vi "TTM.vi"() -> ()   [LabVIEW 2019]
doc: "This is the Target Temperature Monitoring module (TTM).\nIts job is to read all temperature measurement devices and report back the information."
uses:
  TTM Global.vi
panel:
  out "status_THCD401":bool
  in  "port_THCD401":u16=10003
  in  "addr_THCD401":string="192.168.24.17"
  in  "read_flow":bool=TRUE caption="Read Flow"
  out "status_1000":bool
  in  "port_1000":u16=10001
  out "status_He3":bool
  in  "port_He3":u16=10002
  in  "addr_He3":string="192.168.24.17"
  in  "port":u16=10000
  in  "addr":string="192.168.24.17"
  out "status":bool
  in  "Read LakeShore":bool
  in  "Read ITC4":bool
  in  "Read He4 Manometer":bool=TRUE
  in  "Read He3 Manometer":bool
  in  "He4 Range":enum32{"X 1", "X 0.1", "X 0.01", "X 0.001"}(ring)=enum."X 0.01"
  in  "He3 Range":i32(ring)=2 items=["range X0.01", "range X0.1", "range X1"]
  out "TTM Message Type":T1(ring)=enum."He3Range="
  # "He4:100"
  # "He4:1000"
  # "He3"
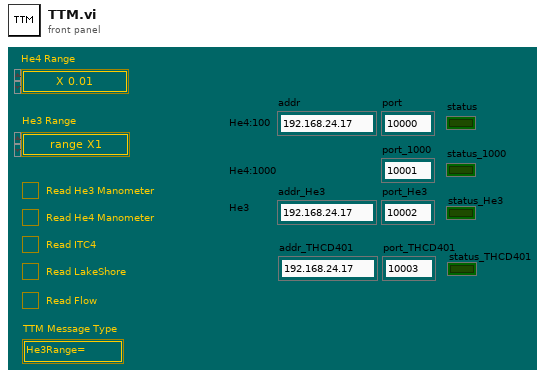
[diagram p1: front panel]
types:
  T1 = enum16{"No Message", "Bad Message", "He3Range=", "He4Range=", "GenEvent=", "Ping=", "Stop"}
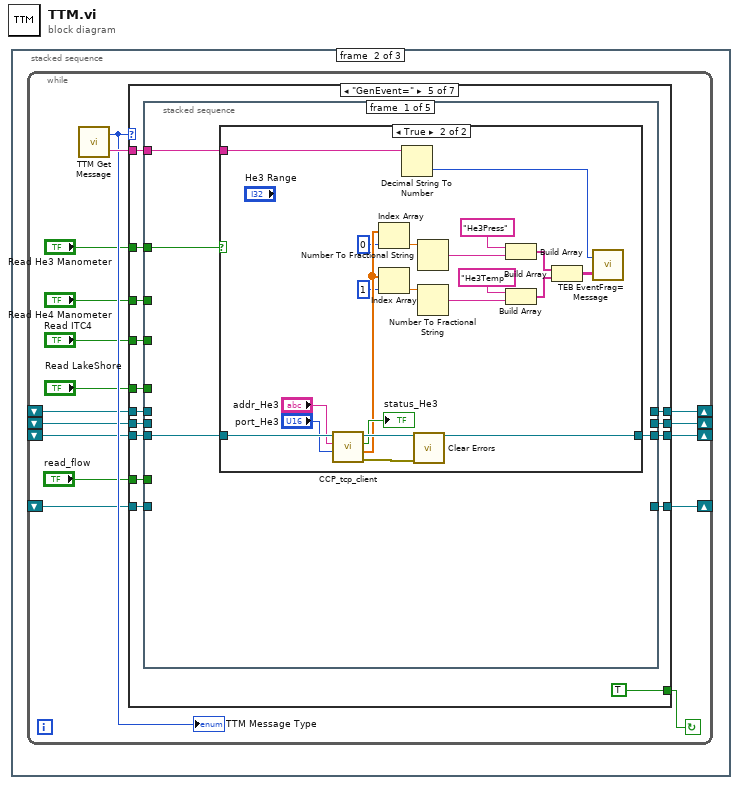
[diagram p0: block diagram]
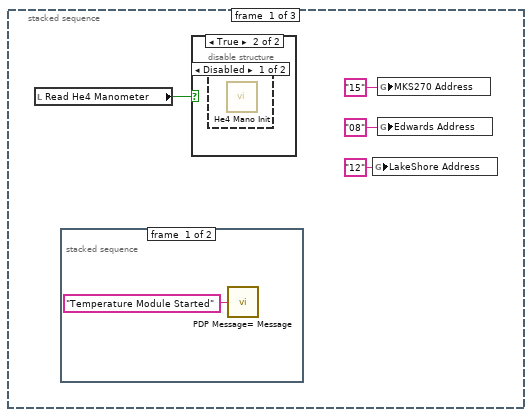
[diagram p2: hidden frame]
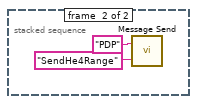
[diagram p5: hidden frame]
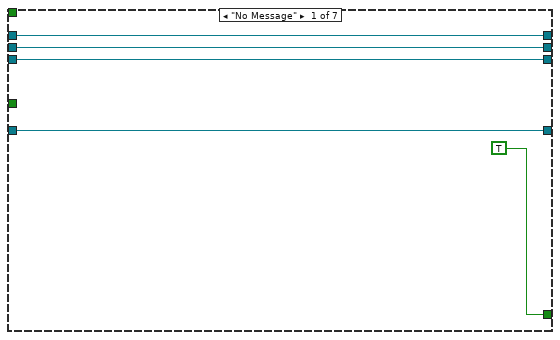
[diagram p6: hidden frame]
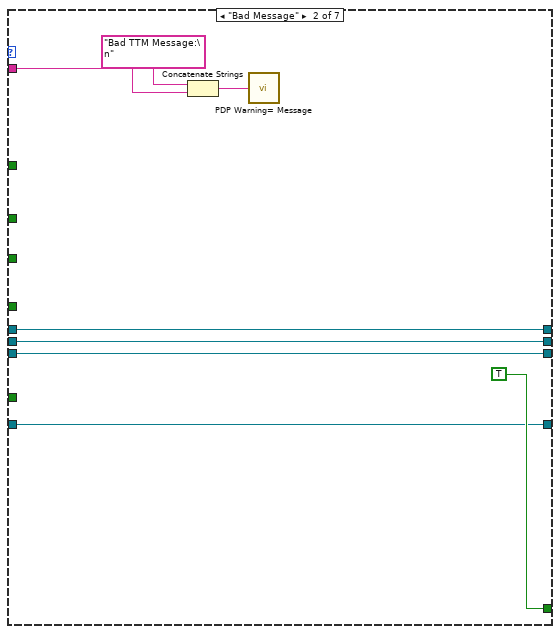
[diagram p7: hidden frame]
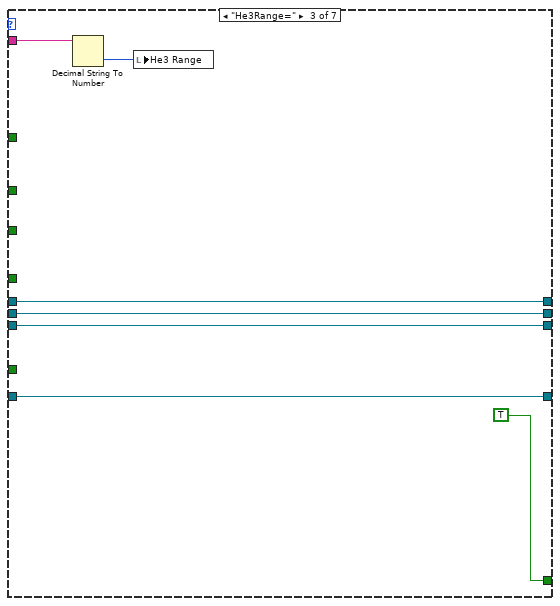
[diagram p8: hidden frame]
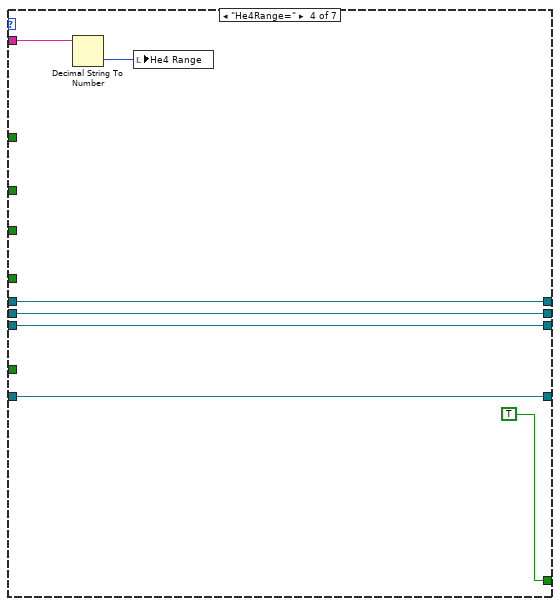
[diagram p9: hidden frame]
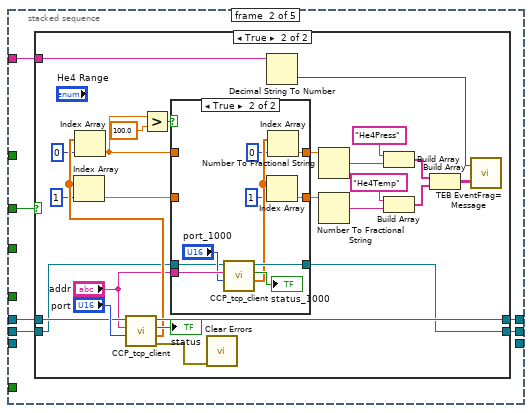
[diagram p11: hidden frame]
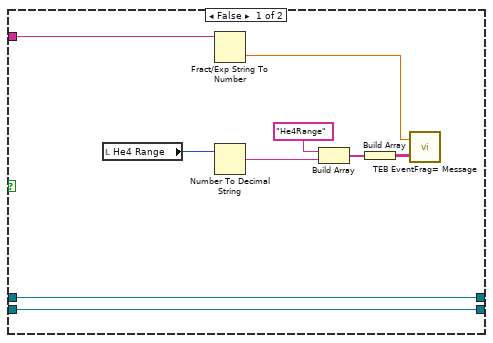
[diagram p12: hidden frame]
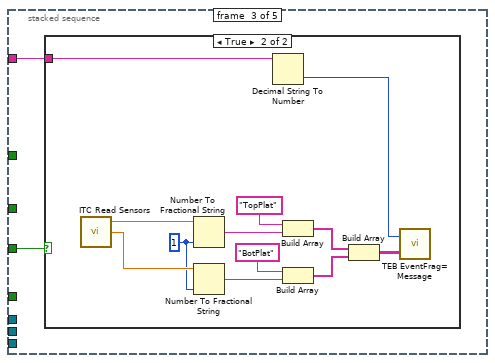
[diagram p14: hidden frame]
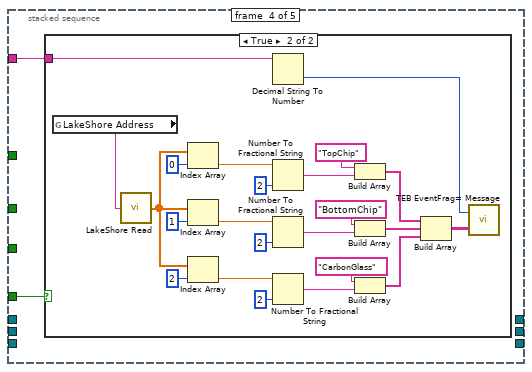
[diagram p16: hidden frame]
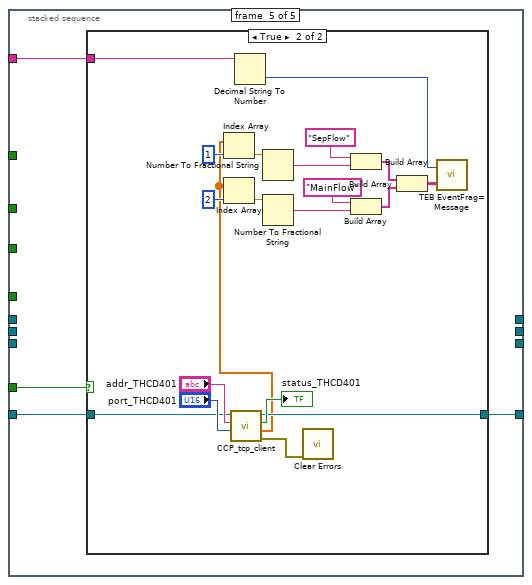
[diagram p18: hidden frame]
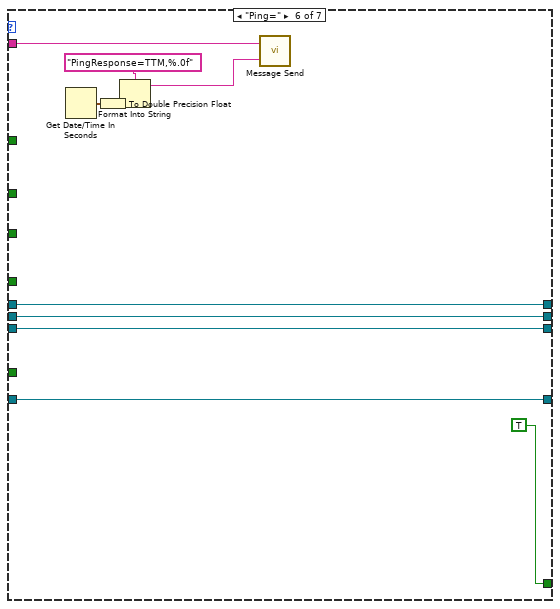
[diagram p20: hidden frame]
diagram:
  n1 = stacked-sequence {
    frame #0 {
      n2 = local read "Read He4 Manometer"() -> (w1:bool)
      n3 = stacked-sequence {
        frame #0 {
          n4 = call "PDP Message= Message.vi"("Message"="Temperature Module Started") -> ()
        }
        frame #1 {
          n5 = call "Message Send.vi"("Message"="SendHe4Range", "Destination"="PDP") -> ()
        }
      }
      n6 = case shown="True" w1 {
        frame False {
        }
        frame True {
          n7 = disable-structure shown="Disabled" {
            frame Disabled {
              n8 = call "He4 Mano Init.vi"() -> ()  [unwired: 1 in]
            }
            frame Enabled {
            }
          }
        }
      }
      n9 = global write "TTM Global.vi" "LakeShore Address"("12" ("Edwards Address")) -> ()
      n10 = global write "TTM Global.vi" "MKS270 Address"("15" ("MKS270 Address")) -> ()
      n11 = global write "TTM Global.vi" "Edwards Address"("08" ("Edwards Address")) -> ()
    }
    frame #1 {
      n12 = while {
        shift-right: [w16] -> _
        shift-left: _ -> [w15]
        shift-right: [w14] -> _
        shift-left: _ -> [w13]
        shift-right: [w12] -> _
        shift-left: _ -> [w11]
        shift-right: [w8] -> _
        shift-left: _ -> [w9]
        stop <- w22 continue-if-true
        n13 = call "TTM Get Message.vi"() -> ("Text"=w23:string, "TTM Message Type"=w21:T1)
        "TTM Message Type" <- w21
        n14 = case shown="\"GenEvent=\"" w21 {
          tunnel: w23 -> [_ w36 w42 w49 w65 w214 _]
          tunnel: [TRUE TRUE TRUE TRUE TRUE TRUE FALSE] -> w22
          tunnel: "Read He3 Manometer" -> [_ _ _ _ w63 _ _]
          tunnel: "Read He4 Manometer" -> [_ _ _ _ w62 _ _]
          tunnel: "Read ITC4" -> [_ _ _ _ w61 _ _]
          tunnel: "Read LakeShore" -> [_ _ _ _ w60 _ _]
          tunnel: [w27 w32 w40 w47 w59 w212 w222] -> w16
          tunnel: w15 -> [w27 w32 w40 w47 w58 w212 w222]
          tunnel: [w26 w31 w39 w46 w57 w211 w221] -> w14
          tunnel: w13 -> [w26 w31 w39 w46 w56 w211 w221]
          tunnel: [w25 w30 w38 w45 w55 w210 w220] -> w12
          tunnel: w11 -> [w25 w30 w38 w45 w54 w210 w220]
          tunnel: "read_flow" -> [_ _ _ _ w53 _ _]
          tunnel: w9 -> [w24 w29 w37 w44 w52 w209 w219]
          tunnel: [w24 w29 w37 w44 w51 w209 w219] -> w8
          frame "No Message" {
          }
          frame "Bad Message" {
            n15 = Concatenate Strings("Bad TTM Message:\n", w36) -> (w34:string)
            n16 = call "PDP Warning= Message.vi"("Message"=w34) -> ()
          }
          frame "He3Range=" {
            n17 = Decimal String To Number(string=w42) -> (number=w41:i32)  [unwired: 2 in, 1 out]
            n18 = local write "He3 Range"(w41) -> ()
          }
          frame "He4Range=" {
            n19 = Decimal String To Number(string=w49) -> (number=w48:i32)  [unwired: 2 in, 1 out]
            n20 = local write "He4 Range"(w48) -> ()
          }
          frame "GenEvent=" {
            n21 = stacked-sequence {
              tunnel: w65 -> [w69 w96 w146 w160 w184]
              tunnel: w63 -> [w68 _ _ _ _]
              tunnel: w62 -> [_ w95 _ _ _]
              tunnel: w61 -> [_ _ w145 _ _]
              tunnel: w60 -> [_ _ _ w159 _]
              tunnel: [_ w94 _ _ _] -> w59
              tunnel: w58 -> [_ w93 _ _ _]
              tunnel: [w67 _ _ _ _] -> w57
              tunnel: w56 -> [w66 _ _ _ _]
              tunnel: [_ w92 _ _ _] -> w55
              tunnel: w54 -> [_ w91 _ _ _]
              tunnel: w53 -> [_ _ _ _ w187]
              tunnel: w52 -> [_ _ _ _ w186]
              tunnel: [_ _ _ _ w185] -> w51
              frame #0 {
                n22 = case shown="True" w68 {
                  tunnel: w69 -> [_ w90]
                  tunnel: [w70 w80] -> w67
                  tunnel: w66 -> [w70 w79]
                  frame False {
                  }
                  frame True {
                    n23 = call "CCP_tcp_client.vi"("port"="port_He3", "address"="addr_He3", "conn_id_in"=w79) -> ("error out"=w81:errorcluster, "array_value"=w75:dbl[], "status"=→"status_He3":bool, "conn_id_out"=w80:refnum<k5>)  [unwired: 5 in]
                    n24 = Index Array(array=w75, index=0) -> (element=w74:dbl)
                    n25 = Index Array(array=w75, index=1) -> (element=w73:dbl)
                    n26 = Decimal String To Number(string=w90) -> (number=w89:i32)  [unwired: 2 in, 1 out]
                    n27 = call <vilib>:"Clear Errors.vi"("error in (no error)"=w81) -> ()  [unwired: 5 in, 2 out]
                    n28 = Number To Fractional String(number=w74) -> (F-format string=w82:string)  [unwired: 3 in]
                    n29 = Number To Fractional String(number=w73) -> (F-format string=w86:string)  [unwired: 3 in]
                    n30 = Build Array("He3Press", w82) -> (w83:string[])
                    n31 = Build Array("He3Temp", w86) -> (w87:string[])
                    n32 = Build Array(w83, w87) -> (w88:string[][])
                    n33 = call "TEB EventFrag= Message.vi"("Event Fragment(s)"=w88, "Event Number"=w89) -> ()
                  }
                }
              }
              frame #1 {
                n34 = case shown="True" w95 {
                  tunnel: w96 -> [w102 w131]
                  tunnel: [w98 w120] -> w94
                  tunnel: w93 -> [w98 w119]
                  tunnel: [w97 w107] -> w92
                  tunnel: w91 -> [w97 w106]
                  frame False {
                    n35 = local read "He4 Range"() -> (w100:enum32{"X 1", "X 0.1", "X 0.01", "X 0.001"})
                    n36 = Fract/Exp String To Number(string=w102) -> (number=w103:dbl)  [unwired: 3 in, 1 out]
                    n37 = Number To Decimal String(number=w100) -> (decimal integer string=w99:string)  [unwired: 1 in]
                    n38 = Build Array("He4Range", w99) -> (w105:string[])
                    n39 = Build Array(w105) -> (w101:string[][])
                    n40 = call "TEB EventFrag= Message.vi"("Event Fragment(s)"=w101, "Event Number"=w103) -> ()
                  }
                  frame True {
                    n41 = call "CCP_tcp_client.vi"("port"="port", "address"="addr", "conn_id_in"=w119) -> ("error out"=w115:errorcluster, "array_value"=w118:dbl[], "status"=→"status":bool, "conn_id_out"=w120:refnum<k5>)  [unwired: 5 in]
                    n42 = Index Array(array=w118, index=1) -> (element=w109:dbl)
                    n43 = Index Array(array=w118, index=0) -> (element=w111:dbl)
                    n44 = Greater?(x=w111, y=100.0) -> (0:w113:bool)
                    n45 = case shown="True" w113 {
                      tunnel: [w134 w139] -> w112
                      tunnel: w111 -> [w134 _]
                      tunnel: [w133 w138] -> w110
                      tunnel: w109 -> [w133 _]
                      tunnel: "addr" -> [_ w144]
                      tunnel: w106 -> [w132 w142]
                      tunnel: [w132 w141] -> w107
                      frame False {
                      }
                      frame True {
                        n46 = call "CCP_tcp_client.vi"("port"="port_1000", "address"=w144, "conn_id_in"=w142) -> ("array_value"=w137:dbl[], "status"=→"status_1000":bool, "conn_id_out"=w141:refnum<k5>)  [unwired: 5 in, 1 out]
                        n47 = Index Array(array=w137, index=1) -> (element=w138:dbl)
                        n48 = Index Array(array=w137, index=0) -> (element=w139:dbl)
                      }
                    }
                    n49 = call <vilib>:"Clear Errors.vi"("error in (no error)"=w115) -> ()  [unwired: 5 in, 2 out]
                    n50 = Decimal String To Number(string=w131) -> (number=w130:i32)  [unwired: 2 in, 1 out]
                    n51 = Number To Fractional String(number=w112) -> (F-format string=w123:string)  [unwired: 3 in]
                    n52 = Number To Fractional String(number=w110) -> (F-format string=w127:string)  [unwired: 3 in]
                    n53 = Build Array("He4Press", w123) -> (w124:string[])
                    n54 = Build Array("He4Temp", w127) -> (w128:string[])
                    n55 = Build Array(w124, w128) -> (w129:string[][])
                    n56 = call "TEB EventFrag= Message.vi"("Event Fragment(s)"=w129, "Event Number"=w130) -> ()
                  }
                }
              }
              frame #2 {
                n57 = case shown="True" w145 {
                  tunnel: w146 -> [_ w158]
                  frame False {
                  }
                  frame True {
                    w147 = i16 1 ("precision (6)")
                    n58 = call "ITC Read Sensors.vi"() -> ("Sensor 2"=w149:dbl, "Sensor 1"=w148:dbl)  [unwired: 1 in]
                    n59 = Number To Fractional String(number=w148, precision (6)=w147) -> (F-format string=w151:string)  [unwired: 2 in]
                    n60 = Number To Fractional String(number=w149, precision (6)=w147) -> (F-format string=w150:string)  [unwired: 2 in]
                    n61 = Decimal String To Number(string=w158) -> (number=w157:i32)  [unwired: 2 in, 1 out]
                    n62 = Build Array("TopPlat", w151) -> (w153:string[])
                    n63 = Build Array("BotPlat", w150) -> (w152:string[])
                    n64 = Build Array(w153, w152) -> (w156:string[][])
                    n65 = call "TEB EventFrag= Message.vi"("Event Fragment(s)"=w156, "Event Number"=w157) -> ()
                  }
                }
              }
              frame #3 {
                n66 = case shown="True" w159 {
                  tunnel: w160 -> [_ w183]
                  frame False {
                  }
                  frame True {
                    n67 = global read "TTM Global.vi" "LakeShore Address"() -> (w165:string)
                    n68 = call "LakeShore Read.vi"("Address"=w165) -> ("subarray"=w164:dbl[])
                    n69 = Index Array(array=w164, index=0) -> (element=w178:dbl)
                    n70 = Index Array(array=w164, index=1) -> (element=w174:dbl)
                    n71 = Index Array(array=w164, index=2) -> (element=w173:dbl)
                    n72 = Decimal String To Number(string=w183) -> (number=w182:i32)  [unwired: 2 in, 1 out]
                    n73 = Number To Fractional String(number=w178, precision (6)=i16 2) -> (F-format string=w176:string)  [unwired: 2 in]
                    n74 = Number To Fractional String(number=w174, precision (6)=i16 2) -> (F-format string=w169:string)  [unwired: 2 in]
                    n75 = Number To Fractional String(number=w173, precision (6)=i16 2) -> (F-format string=w168:string)  [unwired: 2 in]
                    n76 = Build Array("TopChip", w176) -> (w179:string[])
                    n77 = Build Array("BottomChip", w169) -> (w166:string[])
                    n78 = Build Array("CarbonGlass", w168) -> (w167:string[])
                    n79 = Build Array(w179, w166, w167) -> (w181:string[][])
                    n80 = call "TEB EventFrag= Message.vi"("Event Fragment(s)"=w181, "Event Number"=w182) -> ()
                  }
                }
              }
              frame #4 {
                n81 = case shown="True" w187 {
                  tunnel: w186 -> [w188 w205]
                  tunnel: [w188 w204] -> w185
                  tunnel: w184 -> [_ w202]
                  frame False {
                  }
                  frame True {
                    n82 = call "CCP_tcp_client.vi"("port"="port_THCD401", "address"="addr_THCD401", "conn_id_in"=w205) -> ("error out"=w203:errorcluster, "array_value"=w190:dbl[], "status"=→"status_THCD401":bool, "conn_id_out"=w204:refnum<k5>)  [unwired: 5 in]
                    n83 = Index Array(array=w190, index=1) -> (element=w195:dbl)
                    n84 = Index Array(array=w190, index=2) -> (element=w194:dbl)
                    n85 = Decimal String To Number(string=w202) -> (number=w189:i32)  [unwired: 2 in, 1 out]
                    n86 = Number To Fractional String(number=w195) -> (F-format string=w196:string)  [unwired: 3 in]
                    n87 = Number To Fractional String(number=w194) -> (F-format string=w200:string)  [unwired: 3 in]
                    n88 = call <vilib>:"Clear Errors.vi"("error in (no error)"=w203) -> ()  [unwired: 5 in, 2 out]
                    n89 = Build Array("SepFlow", w196) -> (w197:string[])
                    n90 = Build Array("MainFlow", w200) -> (w201:string[])
                    n91 = Build Array(w197, w201) -> (w191:string[][])
                    n92 = call "TEB EventFrag= Message.vi"("Event Fragment(s)"=w191, "Event Number"=w189) -> ()
                  }
                }
              }
            }
          }
          frame "Ping=" {
            n93 = Get Date/Time In Seconds() -> (seconds since 1Jan1904=w213:timestamp)
            n94 = To Double Precision Float(number=w213) -> (double precision float=w216:dbl)
            n95 = Format Into String(format string="PingResponse=TTM,%.0f", w216) -> (resulting string=w215:string)  [unwired: 2 in, 1 out]
            n96 = call "Message Send.vi"("Message"=w215, "Destination"=w214) -> ()
          }
          frame "Stop" {
          }
        }
      }
    }
    frame #2 {
    }
  }
